vi "Update Drag-Drop Visible Steps.vi"(9 "Step Number":i32, 10 "Number of Sequence Steps":i32, 11 "TreeControl in":refnum<vi>) -> ()   [LabVIEW 2020, in "Output Sequencer.lvlib" / "Settings UI.lvclass"]
uses:
  Settings UI.lvclass
  Types/Tree Index Enum.ctl
  Globals/Global Tree Data.vi
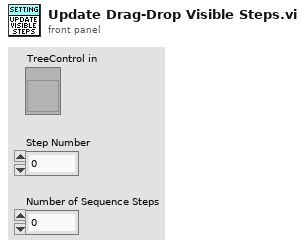
[diagram p1: front panel]
types:
  T1 = typedef "Output Sequencer.lvlib/Settings UI.lvclass/Tree Index Enum.ctl" = enum16{"General Settings", "Num Steps", "Num Analog", "Num Digital", "Show Confirmation", "Interp Priority", "Adv Timing", "Enable Conditions", "Seq Execution", "Reset Test Start", "Only When Test", "Delay After Test", "Start condition", "Re-triggering", "Stop condition", "Stop After Cycles", "Stop Values", "Default Values", "Default Analog", "Default Digital", "Steps", "Step #", "Description", "Precondition", "Duration", "Mode", "Delay Between Vals", "Analog Values", "Digital Values", "Postcondition", "On True", "On False"}
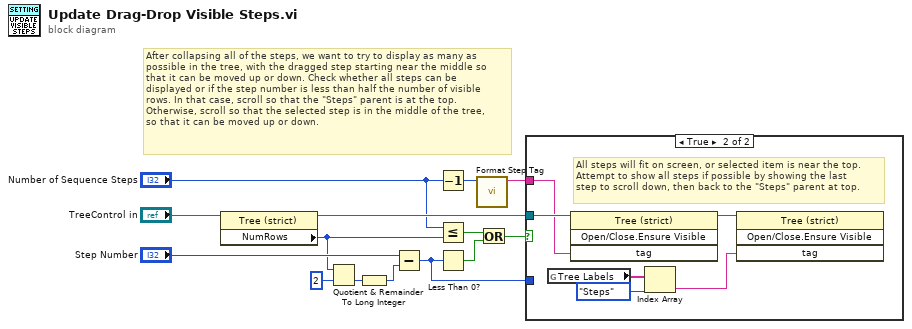
[diagram p0: block diagram]
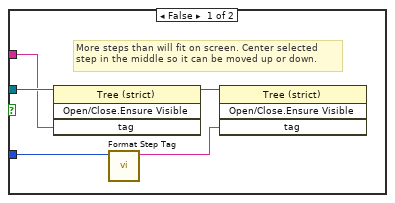
[diagram p2: hidden frame]
diagram:
  # "After collapsing all of the steps, we want to try to display as many as\npossible in the tree, with the dragged step starting near the middle so\nthat it can be moved up or down. Check whether all steps can be\ndisplayed or if the step number is less than half the number of visible\nrows. In that case, scroll so that the \"Steps\" parent is at the top.\nOtherwise, scroll so that the selected step is in the middle of the tree,\nso that it can be moved up or down."
  n1 = property class="Tree (strict)"(reference="TreeControl in") -> (reference out=w12:refnum<vi>, "NumRows"=w3:u32)  [unwired: 1 in, 1 out]
  n2 = Quotient & Remainder(x=w3, y=2) -> (floor(x/y)=w5:u32)  [unwired: 1 out]
  n3 = To Long Integer(number=w5) -> (32bit integer=w4:i32)
  n4 = Subtract(x="Step Number", y=w4) -> (x-y=w9:i32)
  n5 = Decrement(x="Number of Sequence Steps") -> (x-1=w13:i32)
  n6 = Less Or Equal?(x="Number of Sequence Steps", y=w3) -> (x <= y?=w2:bool)
  n7 = Less Than 0?(x=w9) -> (x < 0?=w1:bool)
  n8 = call "Format Step Tag.vi"("Step Number"=w13) -> ("Tag"=w14:string)  [unwired: 10 in]
  n9 = Or(x=w2, y=w1) -> (x .or. y?=w8:bool)
  n10 = case shown="True" w8 {
    tunnel: w14 -> [w15 w20]
    tunnel: w12 -> [w19 w25]
    tunnel: w9 -> [w17 _]
    frame False {
      # "More steps than will fit on screen. Center selected\nstep in the middle so it can be moved up or down."
      n11 = invoke class="Tree (strict)" method="Open/Close.Ensure Visible"(reference=w19, "tag"=w15) -> (reference out=w18:refnum<vi>)  [unwired: 2 in, 3 out]
      n12 = call "Format Step Tag.vi"("Step Number"=w17) -> ("Tag"=w16:string)  [unwired: 10 in]
      n13 = invoke class="Tree (strict)" method="Open/Close.Ensure Visible"(reference=w18, "tag"=w16) -> ()  [unwired: 2 in, 4 out]
    }
    frame True {
      # "All steps will fit on screen, or selected item is near the top.\nAttempt to show all steps if possible by showing the last\nstep to scroll down, then back to the \"Steps\" parent at top."
      n14 = global read "Global Tree Data.vi" "Tree Labels"() -> (w23:string[])
      n15 = invoke class="Tree (strict)" method="Open/Close.Ensure Visible"(reference=w25, "tag"=w20) -> (reference out=w24:refnum<vi>)  [unwired: 2 in, 3 out]
      n16 = Index Array(array=w23, index=Tree_Index_Enum."Steps" ("Tree Index Enum")) -> (element=w21:string)
      n17 = invoke class="Tree (strict)" method="Open/Close.Ensure Visible"(reference=w24, "tag"=w21) -> ()  [unwired: 2 in, 4 out]
    }
  }
